vi "GenerateFlow.vi"(0 "object in":refnum<class "CetoniPump.lvclass">, 2 "Flow Rate":dbl, 5 "error in (no error)":errorcluster) -> (14 "object out":refnum<class "CetoniPump.lvclass">, 19 "error out":errorcluster)   [LabVIEW 2021, in "CetoniPump.lvclass"]
uses:
  CetoniPump.lvclass
  CetoniPump.lvclass/CetoniPump.ctl
  Users/olaja/AppData/Local/CETONI_SDK/lib/labview/labbCAN_Pump_API/labbCAN_Pump_API.lvlib
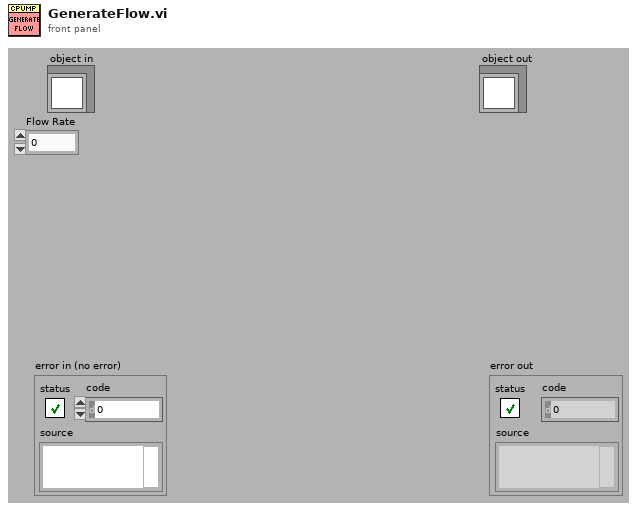
[diagram p1: front panel]
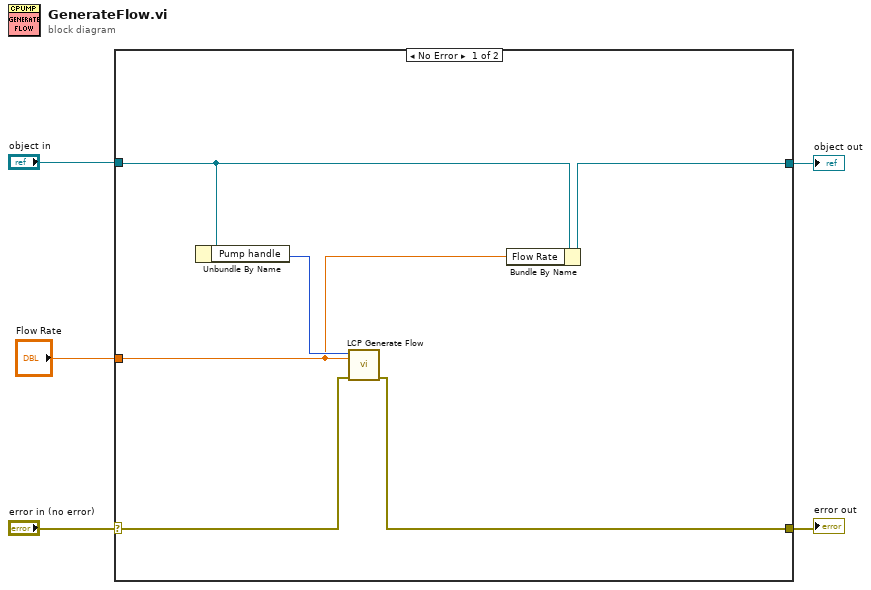
[diagram p0: block diagram]
diagram:
  n1 = case shown="No Error" "error in (no error)" {
    selector: "error in (no error)" -> [w7 w13]
    tunnel: [w6 w13] -> w4
    tunnel: [w10 w12] -> w2
    tunnel: "object in" -> [w11 w12]
    tunnel: "Flow Rate" -> [w8 _]
    frame No Error {
      n2 = Unbundle By Name(w11) -> ("Pump handle"=w9:i64)
      n3 = call "LCP Generate Flow.vi"("error in (no error)"=w7, "Flow Rate"=w8, "Pump Handle"=w9) -> ("error out"=w6:errorcluster)  [unwired: 8 in]
      n4 = Bundle By Name(cluster=w11, "Flow Rate"=w8) -> (w10:refnum<class "CetoniPump.lvclass">)
    }
    frame Error {
    }
  }
  "error out" <- w4
  "object out" <- w2
